vi "Update User.vi"(8 "Error in":errorcluster, 11 "Username":string) -> (0 "Error out":errorcluster)   [LabVIEW 2019, in "User Lib.lvlib"]
uses:
  User Lib.lvlib
  <vilib>/addons/database/Connection.llb/DB Tools Open Connec (String).vi
  <vilib>/addons/database/NI_Database_API.lvlib
  database.lvlib
panel:
  in  "Cancel":bool
  in  "OK":bool
  in  "Is Admin?":enum32{"Yes", "No"}(radio)
  in  "Full Name":string
  out "Username 2":string caption="Username"
  # "Update User"
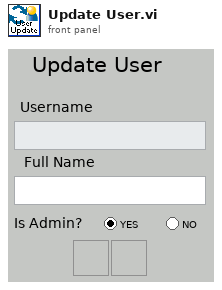
[diagram p1: front panel]
types:
  T1 = typedef "NI_Database_API.lvlib/Conn ObjectReference.ctl" = refnum<k1>
  T2 = cluster{i32, "date/time string":string, "date/time string":string, string}
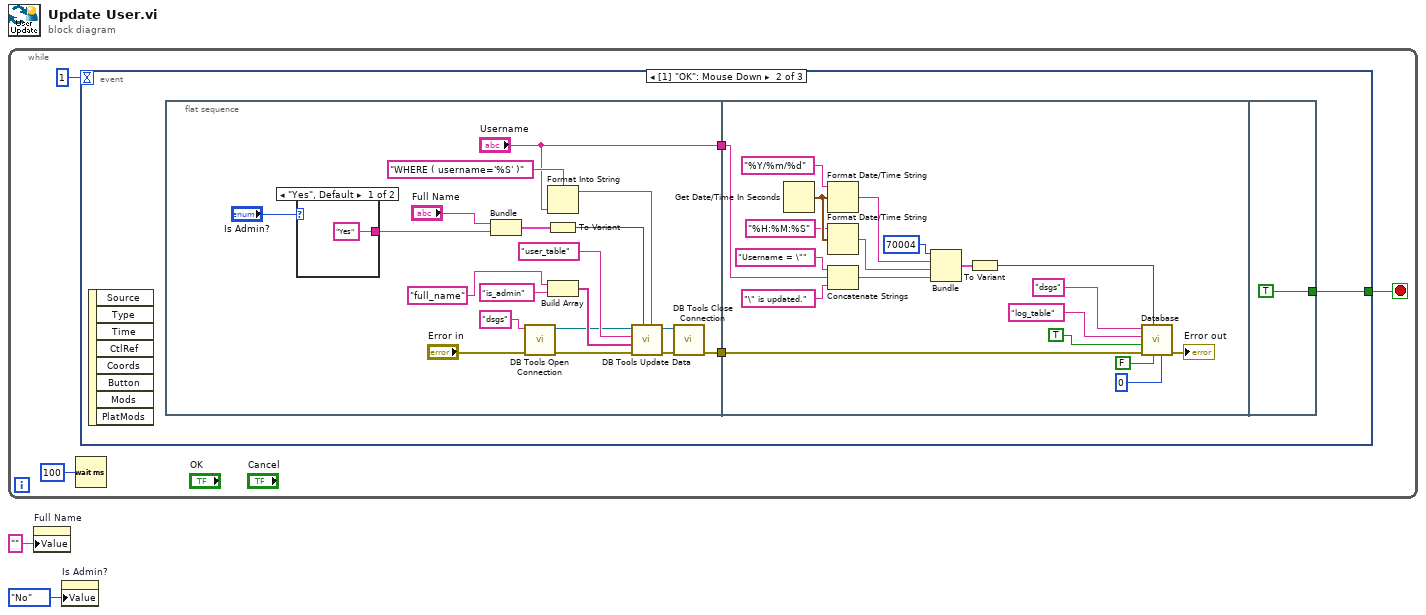
[diagram p0: block diagram]
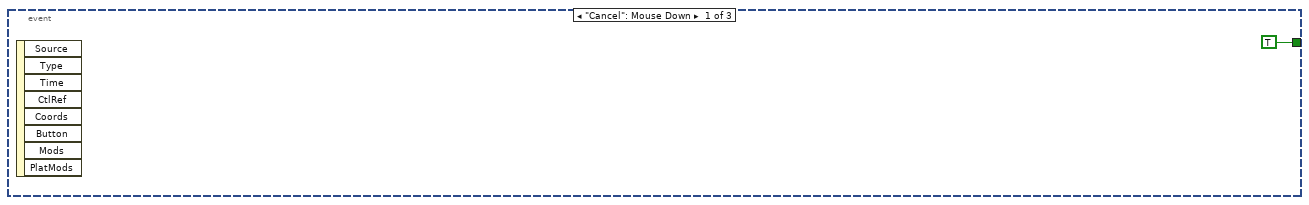
[diagram p2: hidden frame]
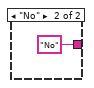
[diagram p3: hidden frame]
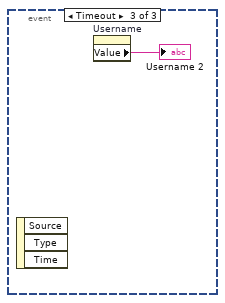
[diagram p4: hidden frame]
diagram:
  n1 = while {
    stop <- w5 stop-if-true
    n2 = Wait (ms)(milliseconds to wait=u32 100) -> ()  [unwired: 1 out]
    n3 = event shown="[1] \"OK\": Mouse Down" {
      selector: _ -> [_ _ _]
      dyn-events: _ -> [_ _ _]
      timeout: 1 -> [_ _ _]
      tunnel: [TRUE w8 _] -> w5
      event "Cancel": Mouse Down {
        n4 = event-data() -> ()  [unwired: 1 in, 8 out]
      }
      event "OK": Mouse Down {
        n5 = event-data() -> ()  [unwired: 1 in, 8 out]
        n6 = flat-sequence {
          tunnel: [w13] -> w9
          tunnel: ["Username"] -> w7
          tunnel: w9 -> [w34]
          tunnel: w7 -> [w32]
          tunnel: [TRUE] -> w8
          frame #0 {
            n7 = case shown="\"Yes\", Default" "Is Admin?" {
              tunnel: ["Yes" ("table") "No" ("table")] -> w25
              frame "Yes", Default {
              }
              frame "No" {
              }
            }
            n8 = Bundle("Full Name"="Full Name", "table"=w25) -> (w15:cluster{"Full Name":string, "table":string})  [unwired: 1 in]
            n9 = call-poly <vilib>:"DB Tools Open Connection.vi"("error in (no error)"="Error in", "connection information"="dsgs") -> ("error out"=w10:errorcluster, "connection reference"=w11:T1)  [unwired: 6 in]
            n10 = Format Into String(format string="WHERE ( username='%S' )" ("condition"), "Username") -> (resulting string=w20:string)  [unwired: 2 in, 1 out]
            n11 = To Variant(anything=w15) -> (Variant=w14:variant)
            n12 = Build Array("full_name" ("table"), "is_admin" ("table")) -> (w18:string[])
            n13 = call <vilib>:"DB Tools Update Data.vi"("condition"=w20, "data"=w14, "error in (no error)"=w10, "columns"=w18, "table"="user_table", "connection reference"=w11) -> ("error out"=w22:errorcluster, "connection reference out"=w21:T1)  [unwired: 4 in]
            n14 = call <vilib>:"DB Tools Close Connection.vi"("error in (no error)"=w22, "connection reference"=w21) -> ("error out"=w13:errorcluster)  [unwired: 5 in]
          }
          frame #1 {
            n15 = Get Date/Time In Seconds() -> (seconds since 1Jan1904=w45:timestamp)
            n16 = Format Date/Time String(time format string (%c)="%Y/%m/%d", seconds (now)=w45) -> (date/time string=w46:string)  [unwired: 1 in]
            n17 = Format Date/Time String(time format string (%c)="%H:%M:%S", seconds (now)=w45) -> (date/time string=w47:string)  [unwired: 1 in]
            n18 = Concatenate Strings("Username = \"" ("string"), w32, "\" is updated." ("string")) -> (w44:string)
            n19 = Bundle(70004, "date/time string"=w46, "date/time string"=w47, w44) -> (w48:T2)  [unwired: 1 in]
            n20 = To Variant(anything=w48) -> (Variant=w49:variant)
            n21 = call "Database.vi"("Maximum Row"=u64 0 ("Storage Time (Day)"), "Delete row?"=FALSE, "Data"=w49, "Error in"=w34, "Auto Increment ID?"=TRUE, "Table"="log_table" ("table"), "Connection"="dsgs" ("table")) -> ("Error out"=→"Error out":errorcluster)  [unwired: 4 in]
          }
          frame #2 {
          }
        }
      }
      event Timeout {
        n22 = event-data() -> ()  [unwired: 1 in, 3 out]
        n23 = property on="Username" class="Str"() -> ("Value"=→"Username 2":string)  [unwired: 2 in, 2 out]
      }
    }
  }
  n24 = property on="Full Name" class="Str"("Value"="" ("Full Name")) -> ()  [unwired: 2 in, 2 out]
  n25 = property on="Is Admin?" class="RadioBtnsControl (strict)"("Value"=enum32{"Yes", "No"}."No" ("Is Admin?")) -> ()  [unwired: 2 in, 2 out]
